vi "Delete Entry.vi"(8 "error in (no error)":errorcluster, 10 "Key":string caption="Name", 11 "Registry in":refnum<class "Registry.lvclass">) -> (0 "error out":errorcluster, 2 "Found?":bool, 3 "Registry out":refnum<class "Registry.lvclass">)   [LabVIEW 2020, in "BCI-1553 API.lvlib" / "Registry.lvlib" / "Registry.lvclass"]
doc: "Deletes a Key/Value pair from the Registry."
uses:
  Registry.lvclass
  Registry.lvclass/Registry.ctl
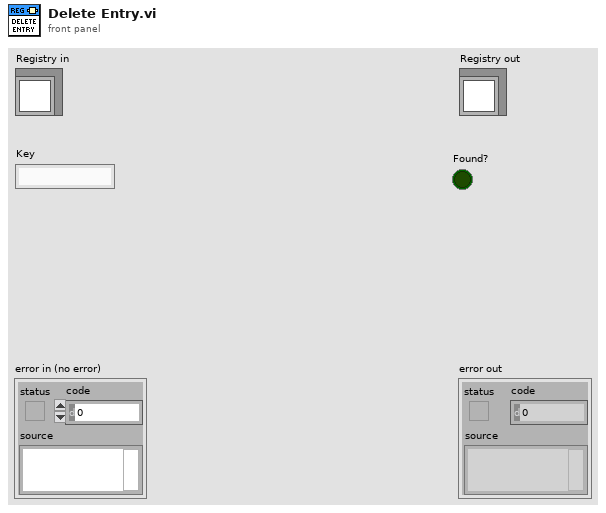
[diagram p1: front panel]
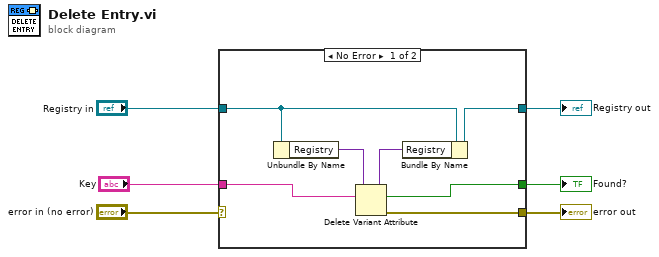
[diagram p0: block diagram]
diagram:
  n1 = case shown="No Error" "error in (no error)" {
    selector: "error in (no error)" -> [_ w15]
    tunnel: [w12 w15] -> w5
    tunnel: [w7 w14] -> w3
    tunnel: "Registry in" -> [w8 w14]
    tunnel: "Key" -> [w13 _]
    tunnel: [w11 _] -> w1
    frame No Error {
      n2 = Unbundle By Name(w8) -> ("Registry"=w10:variant)
      n3 = Delete Variant Attribute(6:w13, 7:w10) -> (0:w12:errorcluster, 2:w11:bool, 3:w9:variant)  [unwired: 1 in]
      n4 = Bundle By Name(cluster=w8, "Registry"=w9) -> (w7:refnum<class "Registry.lvclass">)
    }
    frame Error {
    }
  }
  "error out" <- w5
  "Registry out" <- w3
  "Found?" <- w1
